vi "CalculateXYZ.vi"(1 "CMF":dbl[][](array[numeric]), 2 "Reflectance":dbl[](array[numeric]), 3 "Illuminant":dbl[](array[numeric])) -> (0 "XYZ":dbl[](array[numeric]))   [LabVIEW 2013]
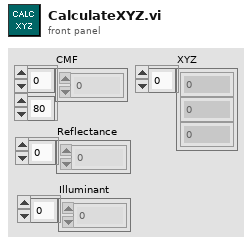
[diagram p1: front panel]
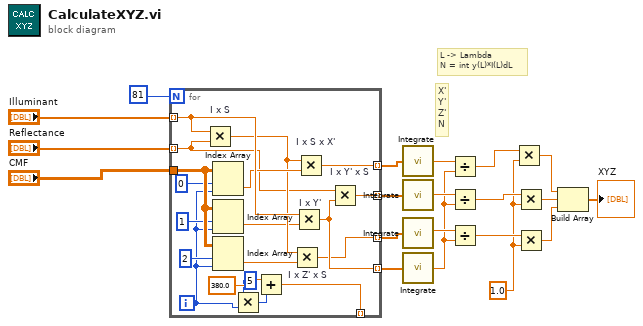
[diagram p0: block diagram]
diagram:
  w8 = 1.0 ("y")
  # "X'\nY'\nZ'\nN"
  # "L -> Lambda\nN = int y(L)*I(L)dL"
  n1 = for {
    N: 81 -> [_]
    tunnel: "CMF" -> [w39]
    tunnel: "Illuminant" -> [w38] mode=indexing
    tunnel: "Reflectance" -> [w34] mode=indexing
    tunnel: [w33] -> w12 mode=indexing
    tunnel: [w32] -> w2 mode=indexing
    tunnel: [w31] -> w3 mode=indexing
    tunnel: [w30] -> w1 mode=indexing
    tunnel: [w21] -> _ mode=indexing
    i -> [w23]
    n2 = Multiply "I x S"(x=w38, y=w34) -> (x*y=w36:dbl)
    n3 = Index Array(array=w39, index (row)=0 ("disabled index (col)"), index (col)=w23) -> (element=w37:dbl)
    n4 = Index Array(array=w39, index (row)=1 ("disabled index (col)"), index (col)=w23) -> (element=w35:dbl)
    n5 = Index Array(array=w39, index (row)=2 ("disabled index (col)"), index (col)=w23) -> (element=w26:dbl)
    n6 = Multiply(x=5, y=w23) -> (x*y=w24:i32)
    n7 = Add(x=380.0, y=w24) -> (x+y=w21:dbl)
    n8 = Multiply "I x Z' x S"(x=w36, y=w26) -> (x*y=w30:dbl)
    n9 = Multiply "I x Y'"(x=w38, y=w35) -> (x*y=w33:dbl)
    n10 = Multiply "I x S x X'"(x=w36, y=w37) -> (x*y=w31:dbl)
    n11 = Multiply "I x Y' x S"(x=w34, y=w33) -> (x*y=w32:dbl)
  }
  n12 = call "Integrate.vi"("Array"=w3) -> ("Integral result"=w19:dbl)
  n13 = call "Integrate.vi"("Array"=w2) -> ("Integral result"=w18:dbl)
  n14 = call "Integrate.vi"("Array"=w1) -> ("Integral result"=w17:dbl)
  n15 = call "Integrate.vi"("Array"=w12) -> ("Integral result"=w16:dbl)
  n16 = Divide(x=w19, y=w16) -> (x/y=w11:dbl)
  n17 = Divide(x=w18, y=w16) -> (x/y=w10:dbl)
  n18 = Divide(x=w17, y=w16) -> (x/y=w9:dbl)
  n19 = Multiply(x=w11, y=w8) -> (x*y=w7:dbl)
  n20 = Multiply(x=w10, y=w8) -> (x*y=w6:dbl)
  n21 = Multiply(x=w9, y=w8) -> (x*y=w5:dbl)
  n22 = Build Array(w7, w6, w5) -> (→"XYZ":dbl[])
